vi "Write InitOptions.vi"(8 "error in (no error)":errorcluster, 10 "InitOptions":T1, 11 "ScopePluginsBase in":refnum<class "ScopePluginsBase.lvclass">) -> (0 "error out":errorcluster, 3 "ScopePluginsBase out":refnum<class "ScopePluginsBase.lvclass">)   [LabVIEW 2018, in "ScopePlugins.lvlib" / "ScopePluginsBase.lvclass"]
uses:
  ScopePluginsBase.lvclass
  TypeDefs/InitializeOptions.ctl
  ScopePluginsBase.lvclass/ScopePluginsBase.ctl
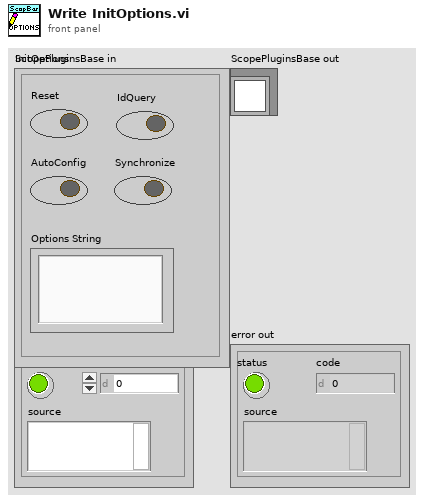
[diagram p1: front panel]
types:
  T1 = typedef "ScopePlugins.lvlib/ScopePluginsBase.lvclass/InitializeOptions.ctl" = cluster{"Reset":bool, "IdQuery":bool, "AutoConfig":bool, "Options String":string, "Synchronize":bool}
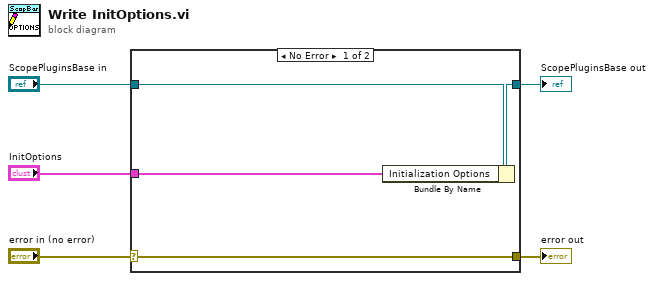
[diagram p0: block diagram]
diagram:
  n1 = case shown="No Error" "error in (no error)" {
    selector: "error in (no error)" -> [w9 w10]
    tunnel: [w9 w10] -> w4
    tunnel: [w7 w11] -> w2
    tunnel: "ScopePluginsBase in" -> [w8 w11]
    tunnel: "InitOptions" -> [w6 _]
    frame No Error {
      n2 = Bundle By Name(cluster=w8, "Initialization Options"=w6) -> (w7:refnum<class "ScopePluginsBase.lvclass">)
    }
    frame Error {
    }
  }
  "error out" <- w4
  "ScopePluginsBase out" <- w2
